vi "Parse ERD Write Expected Data.vi"(0 "Write ERD List":T1[](array[typedef]) {"ERD Number" format="%.0x"}, 11 "Error In":errorcluster) -> (8 "Expected Data":string, 15 "Error Out":errorcluster)   [LabVIEW 2014, in "GEA2_Toolkit.lvlib"]
uses:
  library/GEA2_Toolkit.lvlib
  type defs/ERD Write Data In.ctl
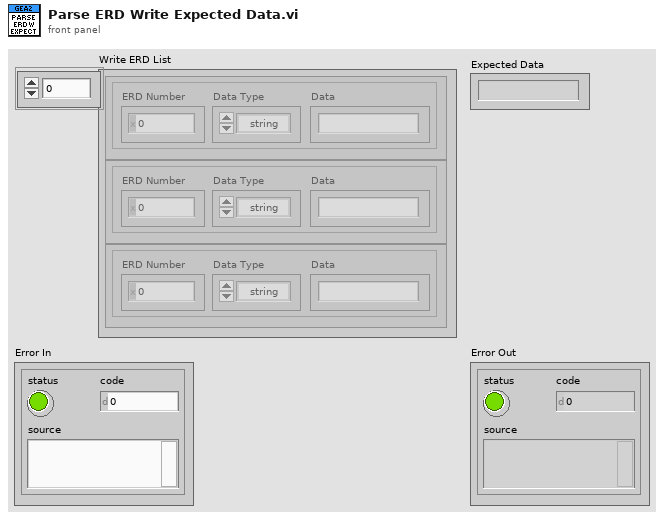
[diagram p1: front panel]
types:
  T1 = typedef "GEA2_Toolkit.lvlib/ERD Write Data In.ctl" = cluster{"ERD Number":u16, "Data Type":enum16{"string", "boolean", "uint8_t", "uint16_t", "uint32_t"}, "Data":string}
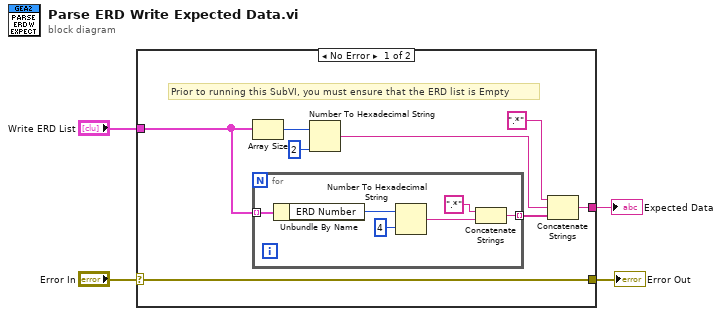
[diagram p0: block diagram]
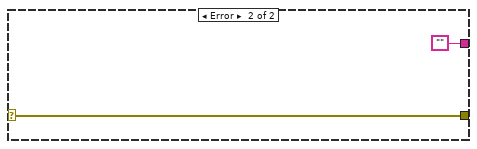
[diagram p2: hidden frame]
diagram:
  n1 = case shown="No Error" "Error In" {
    selector: "Error In" -> [w5 w20]
    tunnel: [w9 ""] -> w4
    tunnel: "Write ERD List" -> [w6 _]
    tunnel: [w5 w20] -> w2
    frame No Error {
      # "Prior to running this SubVI, you must ensure that the ERD list is Empty"
      n2 = Array Size(array=w6) -> (size(s)=w11:i32)
      n3 = for {
        tunnel: w6 -> [w18] mode=indexing
        tunnel: [w13] -> w12 mode=indexing
        n4 = Unbundle By Name(w18) -> ("ERD Number"=w17:u16)
        n5 = Number To Hexadecimal String(1:i16 4 ("width (-)"), 2:w17) -> (0:w15:string)
        n6 = Concatenate Strings(".*" ("string"), w15) -> (w13:string)
      }
      n7 = Number To Hexadecimal String(1:i16 2 ("width (-)"), 2:w11) -> (0:w8:string)
      n8 = Concatenate Strings(".*" ("string"), w8, w12) -> (w9:string)
    }
    frame Error {
    }
  }
  "Expected Data" <- w4
  "Error Out" <- w2
